vi "rmcp_fft.vi"(8 "CP length":u32=64, 9 "fft size":u32=64, 11 "time symbol":cdb[](array[numeric])) -> (3 "freq output":cdb[](array[numeric]))   [LabVIEW 2020]
uses:
  <vilib>/Analysis/2dsp.llb/Complex FFT.vi
  <vilib>/Analysis/NI_AALPro.lvlib
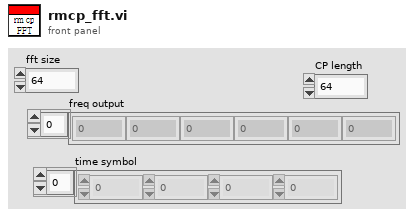
[diagram p1: front panel]
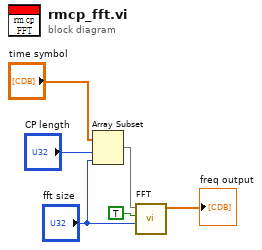
[diagram p0: block diagram]
diagram:
  n1 = Array Subset "Array Subset"(array="time symbol", index="CP length", length="fft size") -> (w4:cdb[])
  n2 = call-poly <vilib>:"FFT.vi"("FFT size"="fft size", "shift?"=TRUE, "X"=w4) -> ("FFT {X}"=→"freq output":cdb[])  [unwired: 7 in, 1 out]
